vi "Go_To_Error_state.vi"(6 "GoTo Error (F)":bool, 8 "Nastêpny stan in":T1=enum."IDLE", 11 "error in (no error)":errorcluster) -> (0 "Nastêpny stan out":T1=enum."IDLE", 3 "error out":errorcluster)   [LabVIEW 2013]
doc: "Przenosi aplikacjê do stanu error w przypadku pojawienia siê b³êdu"
uses:
  inne pliki/Stany.ctl
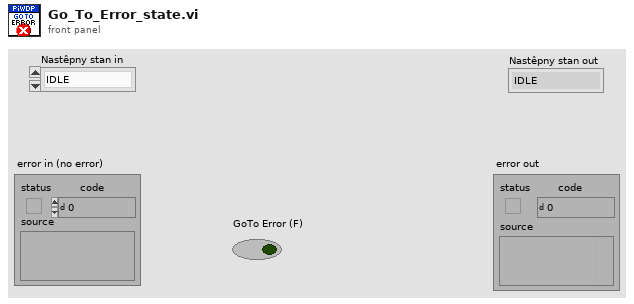
[diagram p1: front panel]
types:
  T1 = typedef "Stany.ctl" = enum16{"Config", "IDLE", "Measure", "Analyze", "Display", "STOP", "Save", "Error", "Error end"}
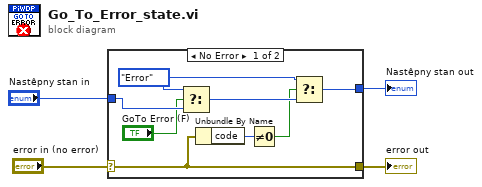
[diagram p0: block diagram]
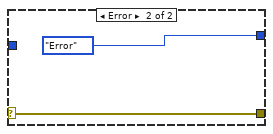
[diagram p2: hidden frame]
diagram:
  n1 = case shown="No Error" "error in (no error)" {
    selector: "error in (no error)" -> [w10 w14]
    tunnel: [w10 w14] -> w3
    tunnel: "Nastêpny stan in" -> [w12 _]
    tunnel: [w7 Stany."Error" ("Nastêpny stan 2")] -> w1
    frame No Error {
      w5 = Stany."Error" ("Nastêpny stan 2")
      n2 = Select(t=w5, s="GoTo Error (F)", f=w12) -> (s? t:f=w8:T1)
      n3 = Unbundle By Name(w10) -> ("code"=w9:i32)
      n4 = Not Equal To 0?(x=w9) -> (x != 0?=w6:bool)
      n5 = Select(t=w5, s=w6, f=w8) -> (s? t:f=w7:T1)
    }
    frame Error {
    }
  }
  "error out" <- w3
  "Nastêpny stan out" <- w1
